vi "Add MVC Actors to Project.vi"   [LabVIEW 2023, in "MVC Actors.lvlib"]
doc: "Run this VI to add the MVC Actors library to the current project"
uses:
  MVC Actors.lvlib
  0ef23a92-ab52-4f24-952a-336d565c94af.vi
panel:
  # "Run this VI to add the MVC Actors Library to the current project"
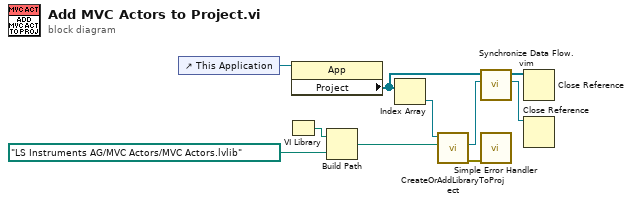
[diagram p0: block diagram]
diagram:
  n1 = control-ref of="This Application"() -> (w10:refnum<vi>)
  n2 = VI Library() -> (path=w8:path)
  n3 = property class="App"(reference=w10) -> ("Project"=w4:refnum<vi>[])  [unwired: 1 in, 2 out]
  n4 = Build Path(base path=w8, name or relative path=path "LS Instruments AG/MVC Actors/MVC Actors.lvlib") -> (appended path=w6:path)
  n5 = Index Array(array=w4) -> (element=w7:refnum<vi>)  [unwired: 1 in]
  n6 = call <vilib>:"CreateOrAddLibraryToProject.vi"("Library Path In (Create New)"=w6, "Project Reference In (Create New)"=w7) -> ("error out"=w2:errorcluster, "Library Reference Out"=w1:refnum<vi>)  [unwired: 7 in, 1 out]
  n7 = call "Synchronize Data Flow.vim"("input 2"=w1, "input 1"=w4) -> ("output 2"=w5:refnum<vi>, "output 1"=w3:refnum<vi>[])  [unwired: 2 in, 2 out]
  n8 = call <vilib>:"Simple Error Handler.vi"("error in (no error)"=w2) -> ()  [unwired: 4 in, 5 out]
  n9 = Close Reference(reference=w3) -> ()  [unwired: 1 in, 1 out]
  n10 = Close Reference(reference=w5) -> ()  [unwired: 1 in, 1 out]
